vi "Check Parameter.vi"(6 "Options in":T1={"DbType"=-1, "Direction"=-1, "Size"=-1, "Precision"=255, "Scale"=255} {"Direction" items=["Input"=1, "Output"=2, "InputOutput"=3, "ReturnValue"=6]; "DbType" items=["AnsiString"=0, "Binary"=1, "Byte"=2, "Boolean"=3, "Currency"=4, "Date"=5, "DateTime"=6, "Decimal"=7, "Double"=8, "Guid"=9, "Int16"=10, "Int32"=11, "Int64"=12, "Object"=13, "SByte"=14, "Single"=15, "String"=16, "Time"=17, "UInt16"=18, "UInt32"=19, "UInt64"=20, "VarNumeric"=21, "AnsiStringFixedLength"=22, "StringFixedLength"=23, "Xml"=25, "DateTime2"=26, "DateTimeOffset"=27]}, 8 "error in (no error)":errorcluster, 9 "value in":variant, 10 "name in":string, 11 "KDBConnection in":refnum<class "DBC.lvclass">) -> (0 "error out":errorcluster, 1 "value out":variant, 2 "name out":string, 3 "KDBConnection out":refnum<class "DBC.lvclass">, 4 "Options out":T1={"DbType"=-1, "Direction"=-1, "Size"=-1, "Precision"=255, "Scale"=255} {"Direction" items=["Input"=1, "Output"=2, "InputOutput"=3, "ReturnValue"=6]; "DbType" items=["AnsiString"=0, "Binary"=1, "Byte"=2, "Boolean"=3, "Currency"=4, "Date"=5, "DateTime"=6, "Decimal"=7, "Double"=8, "Guid"=9, "Int16"=10, "Int32"=11, "Int64"=12, "Object"=13, "SByte"=14, "Single"=15, "String"=16, "Time"=17, "UInt16"=18, "UInt32"=19, "UInt64"=20, "VarNumeric"=21, "AnsiStringFixedLength"=22, "StringFixedLength"=23, "Xml"=25, "DateTime2"=26, "DateTimeOffset"=27]})   [LabVIEW 2020, in "ORM_DBC_Kdb.lvlib" / "DBC.lvclass"]
uses:
  DBC.lvclass
  <vilib>/Viviota/shared/ORM.lvlibp/ORM/DbConnection/DbConnection.lvclass
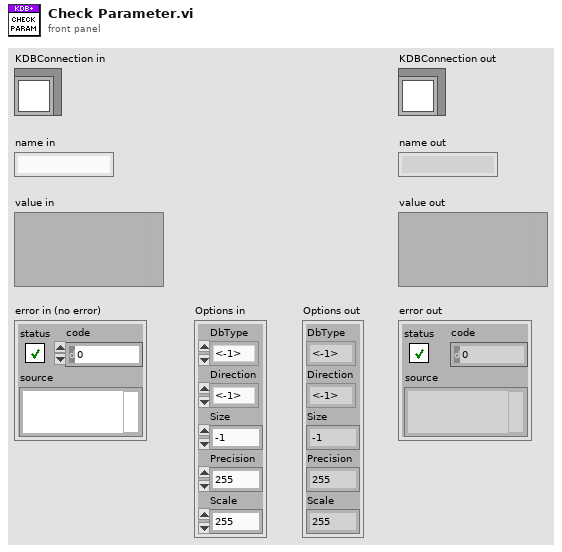
[diagram p1: front panel]
types:
  T1 = cluster{"DbType":i32, "Direction":i32, "Size":i32, "Precision":u8, "Scale":u8}
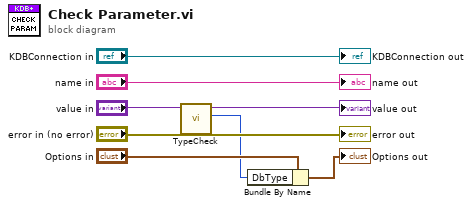
[diagram p0: block diagram]
diagram:
  n1 = call <vilib>:"TypeCheck.vi"("Variant in"="value in") -> ("DbType"=w1:i32, "Variant out"=→"value out":variant)  [unwired: 9 in]
  n2 = Bundle By Name(cluster="Options in", "DbType"=w1) -> (→"Options out":T1)
  "error out" <- "error in (no error)"
  "KDBConnection out" <- "KDBConnection in"
  "name out" <- "name in"
